vi "Smart IO Get Pwm Input.vi"(8 "error in (no error)":errorcluster, 11 "deviceIndex":i32) -> (0 "error out":errorcluster, 1 "period (microsec)":i32, 2 "value (microsec)":i32)   [LabVIEW 2026, in "MrcLib.lvlib"]
doc: "Returns the high time and total period time for the selected device channel assuming it is configured for PWM input operation"
uses:
  MrcLib.lvlib
  Types/MRC Smart IO Mode.ctl
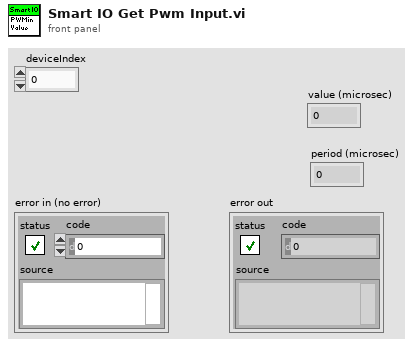
[diagram p1: front panel]
types:
  T1 = typedef "MRC Smart IO Mode.ctl" = i32
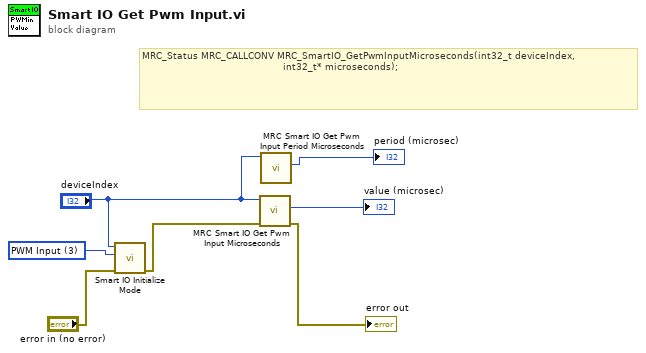
[diagram p0: block diagram]
diagram:
  w1 = T1 3 items=["Digital Input"=0, "Digital Output"=1, "Analog Input"=2, "PWM Input"=3, "PWM Output"=4, "Counter Rising"=5, "Counter Falling"=6, "Addressable LEDs"=13] ("mode")
  # "MRC_Status MRC_CALLCONV MRC_SmartIO_GetPwmInputMicroseconds(int32_t deviceIndex,\n                                               int32_t* microseconds);"
  n1 = call "Smart IO Initialize Mode.vi"("error in (no error)"="error in (no error)", "mode"=w1, "deviceIndex"="deviceIndex") -> ("error out"=w3:errorcluster)  [unwired: 8 in]
  n2 = call "MRC Smart IO Get Pwm Input Microseconds.vi"("error in (no error)"=w3, "deviceIndex"="deviceIndex") -> ("error out"=→"error out":errorcluster, "microseconds out"=→"value (microsec)":i32)  [unwired: 8 in]
  n3 = call "MRC Smart IO Get Pwm Input Period Microseconds.vi"("deviceIndex"="deviceIndex") -> ("microseconds out"=→"period (microsec)":i32)  [unwired: 9 in, 1 out]
